vi "SEK2019v1Giro.vi"(8 "ANGULO":sgl, 9 "NXT/EV3":T1) -> (1 "NXT/EV3 2":T1)   [LabVIEW 2016]
uses:
  <vilib>/NXT/Subs/LVHSConnector.ctl
  <vilib>/NXT/LegoClasses/BrickReference/BrickReference.lvclass
  <vilib>/NXT/Block Support/NXT_OutputPort.ctl
  <vilib>/NXT/Block Support/NXT_InputPort.ctl
  <vilib>/NXT/Dual Mode Library/Sensors/EV3_Gyro_Angle.vi
  <vilib>/NXT/NXTIO Xnodes/NXTIONodeSubVIs/NXTMoveMotors.vi
  <vilib>/NXT/NXTIO Xnodes/NXTIONodeSubVIs/NXTStopMotors.vi
  <vilib>/NXT/NXTIO Xnodes/AddressXNode/NXTIOAddress.xnode
  <vilib>/NXT/NXTIO Xnodes/NXTIOXNode/NXTIO.xnode
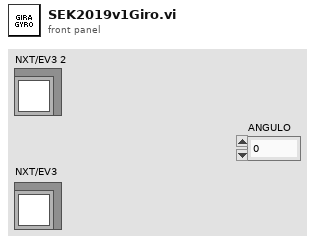
[diagram p1: front panel]
types:
  T1 = typedef "LVHSConnector.ctl" = refnum<class "BrickReference.lvclass">
  T2 = typedef "NXT_InputPort.ctl" = u32
  T3 = typedef "NXT_OutputPort.ctl" = u8
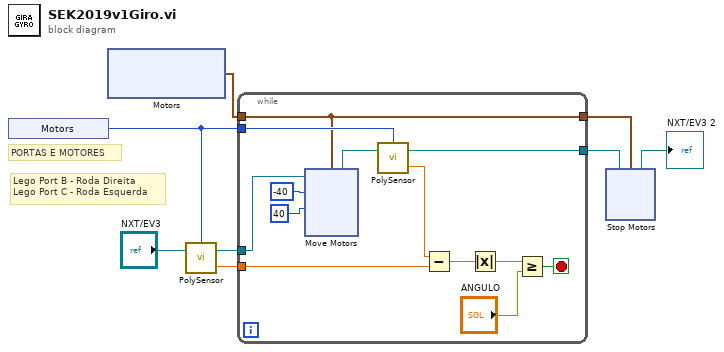
[diagram p0: block diagram]
diagram:
  # "Lego Port B - Roda Direita\nLego Port C - Roda Esquerda"
  # "PORTAS E MOTORES"
  n1 = xnode "Motors"() -> ("Sensor"=w2:T2)
  n2 = xnode "Motors"() -> ("Motor"=w8:cluster{"Port":T3, "Port":T3})
  n3 = call-poly <vilib>:"PolySensor.vi"("NXT/EV3"="NXT/EV3", "Port (Port 1)"=w2) -> ("Degrees"=w1:sgl, "NXT/EV3"=w3:T1)  [unwired: 1 in]
  n4 = while {
    tunnel: w8 -> [w16]
    tunnel: w2 -> [w20]
    tunnel: [w16] -> w6
    tunnel: [w13] -> w4
    tunnel: w3 -> [w9]
    tunnel: w1 -> [w11]
    stop <- w21 stop-if-true
    n5 = xnode "Move Motors"("Power/Speed 2"=i8 40, "Power/Speed 1"=i8 -40, "Motors"=w16, "NXT/EV3"=w9) -> ("NXT/EV3"=w17:T1)
    n6 = call-poly <vilib>:"PolySensor.vi"("NXT/EV3"=w17, "Port (Port 1)"=w20) -> ("Degrees"=w10:sgl, "NXT/EV3"=w13:T1)  [unwired: 1 in]
    n7 = Subtract(x=w10, y=w11) -> (x-y=w12:sgl)
    n8 = Absolute Value(x=w12) -> (abs(x)=w14:sgl)
    n9 = Greater Or Equal?(x=w14, y="ANGULO") -> (x >= y?=w21:bool)
  }
  n10 = xnode "Stop Motors"("Motors"=w6, "NXT/EV3"=w4) -> ("NXT/EV3"=→"NXT/EV3 2":T1)
